vi "Sprach Array leeren Rest stutzen.vi"(11 "Array in":string[][](array[string])) -> (2 "Array entfernt":string[][](array[string]), 3 "Array out":string[][](array[string]))   [LabVIEW 2015, in "Sprachverwaltung.lvlib"]
uses:
  Sprachverwaltung.lvlib
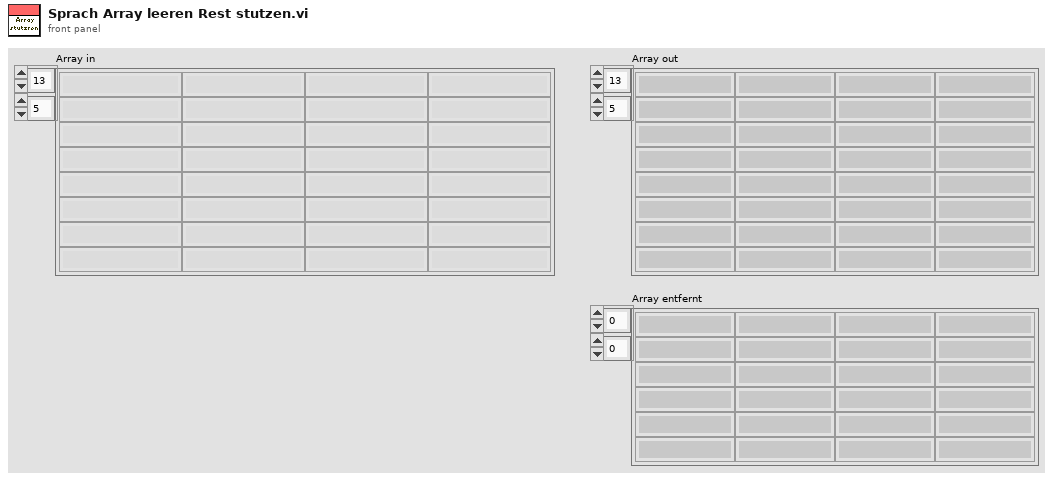
[diagram p1: front panel]
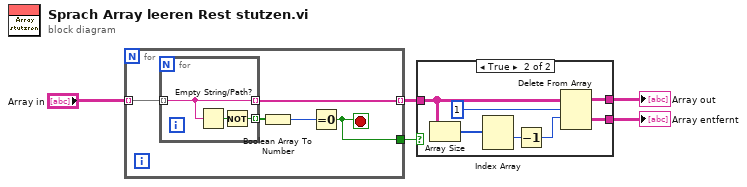
[diagram p0: block diagram]
diagram:
  n1 = for {
    tunnel: "Array in" -> [w10] mode=indexing
    tunnel: [w7] -> w3 mode=indexing
    tunnel: [w6] -> w4
    stop <- w6 stop-if-true
    n2 = for {
      tunnel: w10 -> [w12] mode=indexing
      tunnel: [w11] -> w9 mode=indexing
      tunnel: [w12] -> w7 mode=indexing
      n3 = Empty String/Path?(string/path=w12) -> (empty?=w13:bool)
      n4 = Not(x=w13) -> (.not. x?=w11:bool)
    }
    n5 = Boolean Array To Number(Boolean array=w9) -> (number=w8:u32)
    n6 = Equal To 0?(x=w8) -> (x = 0?=w6:bool)
  }
  n7 = case shown="True" w4 {
    tunnel: w3 -> [w14 w19]
    tunnel: [w14 w18] -> w2
    tunnel: [_ w17] -> w1
    frame False {
    }
    frame True {
      n8 = Array Size(array=w19) -> (size(s)=w20:i32[])
      n9 = Index Array(array=w20) -> (element #1=w16:i32)  [unwired: 2 in, 1 out]
      n10 = Decrement(x=w16) -> (x-1=w15:i32)
      n11 = Delete From Array(array=w19, length=1 ("Länge"), index (row)=w15) -> (deleted portion=w17:string[][], array with subset deleted=w18:string[][])  [unwired: 1 in]
    }
  }
  "Array out" <- w2
  "Array entfernt" <- w1
